vi "Allocate Image Memory.vi"(10 "Base Image File":string, 11 "Reference Image File":string) -> (0 "error out":errorcluster, 1 "Reference Image":T1, 2 "HSL Threshold":T1, 3 "Acquisition Memory":T1[](array[typedef]), 4 "Base Image":T1, 5 "Mask":T1)   [LabVIEW 2018]
uses:
  <vilib>/vision/Image Controls.llb/IMAQ Image.ctl
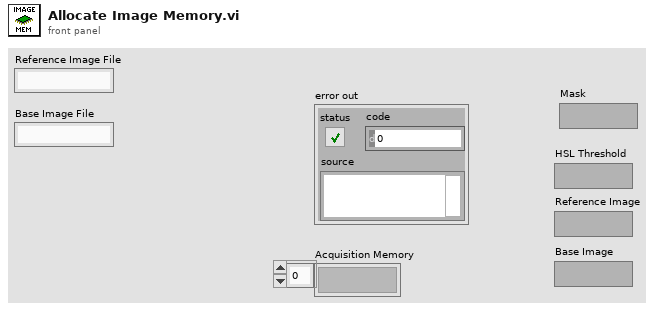
[diagram p1: front panel]
types:
  T1 = typedef "IMAQ Image.ctl" = refnum<image>
  T2 = typedef "Image Type" = u32
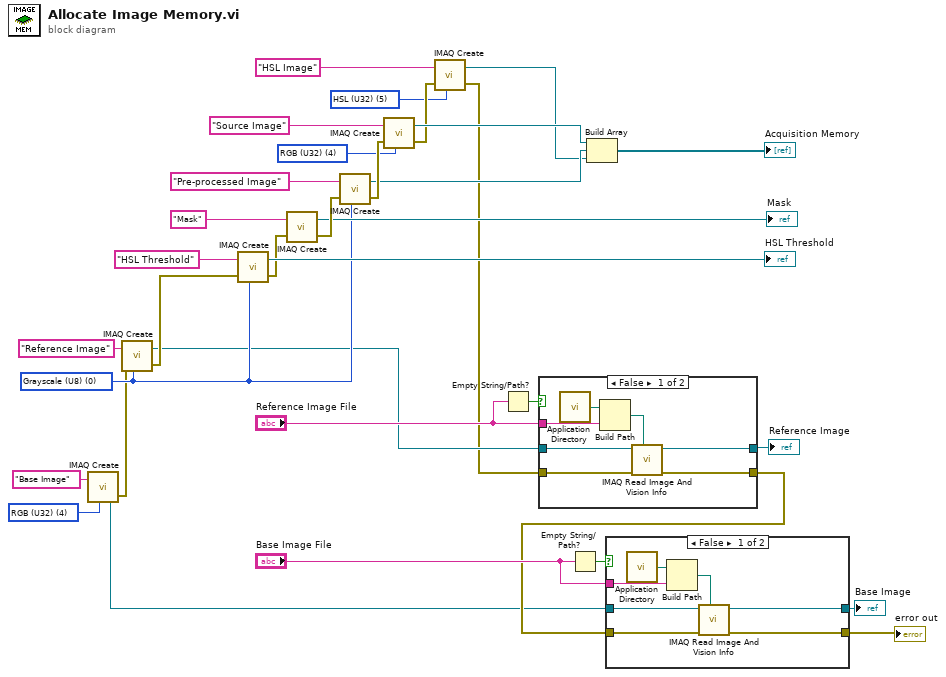
[diagram p0: block diagram]
diagram:
  w1 = T2 5 items=["Grayscale (U8)", "Grayscale (I16)", "Grayscale (SGL)", "Complex (CSG)", "RGB (U32)", "HSL (U32)", "RGB (U64)", "Grayscale (U16)"] ("Image Type")
  w7 = T2 4 items=["Grayscale (U8)", "Grayscale (I16)", "Grayscale (SGL)", "Complex (CSG)", "RGB (U32)", "HSL (U32)", "RGB (U64)", "Grayscale (U16)"] ("Image Type")
  w17 = T2 4 items=["Grayscale (U8)", "Grayscale (I16)", "Grayscale (SGL)", "Complex (CSG)", "RGB (U32)", "HSL (U32)", "RGB (U64)", "Grayscale (U16)"] ("Image Type")
  w16 = T2 0 items=["Grayscale (U8)", "Grayscale (I16)", "Grayscale (SGL)", "Complex (CSG)", "RGB (U32)", "HSL (U32)", "RGB (U64)", "Grayscale (U16)"] ("Image Type")
  n1 = call "IMAQ Create"("Image Name"="Base Image", "Image Type"=w7) -> ("New Image"=w6:T1, "error out"=w8:errorcluster)  [unwired: 3 in]
  n2 = call "IMAQ Create"("Image Name"="Reference Image", "Image Type"=w16, "error in (no error)"=w8) -> ("New Image"=w12:T1, "error out"=w18:errorcluster)  [unwired: 2 in]
  n3 = call "IMAQ Create"("Image Name"="HSL Threshold", "Image Type"=w16, "error in (no error)"=w18) -> ("New Image"=→"HSL Threshold":T1, "error out"=w22:errorcluster)  [unwired: 2 in]
  n4 = call "IMAQ Create"("Image Name"="Mask", "error in (no error)"=w22) -> ("New Image"=→"Mask":T1, "error out"=w21:errorcluster)  [unwired: 3 in]
  n5 = call "IMAQ Create"("Image Name"="Pre-processed Image", "Image Type"=w16, "error in (no error)"=w21) -> ("New Image"=w25:T1, "error out"=w26:errorcluster)  [unwired: 2 in]
  n6 = call "IMAQ Create"("Image Name"="Source Image", "Image Type"=w17, "error in (no error)"=w26) -> ("New Image"=w24:T1, "error out"=w5:errorcluster)  [unwired: 2 in]
  n7 = call "IMAQ Create"("Image Name"="HSL Image", "Image Type"=w1, "error in (no error)"=w5) -> ("New Image"=w2:T1, "error out"=w4:errorcluster)  [unwired: 2 in]
  n8 = Empty String/Path?(string/path="Reference Image File") -> (empty?=w31:bool)
  n9 = case shown="False" w31 {
    tunnel: w12 -> [w39 w43]
    tunnel: "Reference Image File" -> [w38 _]
    tunnel: w4 -> [w37 w42]
    tunnel: [w36 w43] -> w28
    tunnel: [w35 w42] -> w10
    frame False {
      n10 = call <vilib>:"Application Directory.vi"() -> ("Application Directory"=w41:path)
      n11 = Build Path(base path=w41, name or relative path=w38) -> (appended path=w40:path)
      n12 = call "IMAQ Read Image And Vision Info"("File Path"=w40, "error in (no error)"=w37, "Image"=w39) -> ("error out"=w35:errorcluster, "Image Out"=w36:T1)  [unwired: 6 in, 1 out]
    }
    frame True {
    }
  }
  "Reference Image" <- w28
  n13 = Empty String/Path?(string/path="Base Image File") -> (empty?=w15:bool)
  n14 = Build Array(w24, w25, w2) -> (→"Acquisition Memory":T1[])
  n15 = case shown="False" w15 {
    tunnel: w6 -> [w48 w52]
    tunnel: "Base Image File" -> [w47 _]
    tunnel: w10 -> [w46 w51]
    tunnel: [w45 w52] -> w14
    tunnel: [w44 w51] -> w13
    frame False {
      n16 = call <vilib>:"Application Directory.vi"() -> ("Application Directory"=w50:path)
      n17 = Build Path(base path=w50, name or relative path=w47) -> (appended path=w49:path)
      n18 = call "IMAQ Read Image And Vision Info"("File Path"=w49, "error in (no error)"=w46, "Image"=w48) -> ("error out"=w44:errorcluster, "Image Out"=w45:T1)  [unwired: 6 in, 1 out]
    }
    frame True {
    }
  }
  "error out" <- w13
  "Base Image" <- w14
